vi "PSU Limit Check.vi"(8 "Error In":errorcluster, 10 "Supply Output":T1 {"Current mean" format="%.8f"; "Voltage mean" format="%.8f"; "Voltage min" format="%#_8g"; "Voltage max" format="%#_8g"; "Current min" format="%#_8g"; "Current max" format="%#_8g"}, 11 "Config Type":T2={"PSU"={"Current Lower (mA)"=0.0, "Current Upper (mA)"=0.0, "Voltage Lower (V)"=0.0, "Voltage Upper (V)"=0.0}, "Mic"={"Sensitivity (mV/Pa)"={"Lower"=0.0, "Upper"=0.0}, "THD (%)"={"Lower"=0.0, "Upper"=0.0}, "Freq Response"=[]}, "Power Supply"={"Channel Name"="1", "Source Delay (Sec)"=0.5, "Measurement:Sense"=1008, "voltage level"=0.0, "voltage level range"=20.0, "current limit"=0.02, "current limit range"=0.02, "resource name"="PSU"}, "Test Sweep"={"Input Settings"={"IEPE min time to settle [s]"=0.0, "Responce Channel Settings"={"DSA response channel settings"={"coupling"=10045, "enable IEPE excitation"=FALSE, "IEPE current [mA]"=4.0}, "response channel info"={"sensor sensitivity"=1000.0, "engineering units"=1, "dB reference"=1.0, "custom label"="EU", "weighting filter"=0, "pregain"=0.0}, "AI response settings"={"response channel"="SOUNDACQ/ai1", "max value [V]"=10.0, "min value [V]"=-10.0, "terminal configuration"=-1}}, "Stimulus Channel Settings"={"AI stimulus settings"={"stimulus channel"="SOUNDACQ/ai0", "max value [V]"=2.0, "min value [V]"=-2.0, "terminal configuration"=-1}, "DSA stimulus channel settings"={"coupling"=10045, "enable IEPE excitation"=TRUE, "IEPE current [mA]"=4.0}, "stimulus channel info"={"sensor sensitivity"=11.4, "engineering units"=2, "dB reference"=2e-05, "custom label"="EU", "weighting filter"=0, "pregain"=0.0}}}, "Output Settings"={"AO source settings"={"excitation channel"="SOUNDACQ/ao0", "max value [V]"=10.0, "min value [V]"=-10.0, "terminal configuration"=-1}}}} {"Test Sweep"."Output Settings"."AO source settings"."terminal configuration" items=["Default"=-1, "RSE"=10083, "Differential"=10106, "Pseudodifferential"=12529]; "Test Sweep"."Output Settings"."AO source settings"."min value [V]" format="%0.2f"; "Test Sweep"."Output Settings"."AO source settings"."max value [V]" format="%0.2f"; "Test Sweep"."Input Settings"."Stimulus Channel Settings"."stimulus channel info"."pregain" format="%.2f"; "Test Sweep"."Input Settings"."Stimulus Channel Settings"."stimulus channel info"."weighting filter" items=["Linear", "A-weighting", "B-weighting", "C-weighting", "ITU-R 468-4", "Dolby", "CCITT", "C-message", "Wb", "Wc", "Wd", "We", "Wf", "Wh", "Wj", "Wk", "Wm", "AES17 20 kHz lowpass", "AES17 40 kHz lowpass", "AES17 20 kHz highpass", "AES17 40 kHz highpass"]; "Test Sweep"."Input Settings"."Stimulus Channel Settings"."stimulus channel info"."dB reference" format="%^.1e"; "Test Sweep"."Input Settings"."Stimulus Channel Settings"."stimulus channel info"."engineering units" items=["custom..."=0, "V"=1, "A"=21, "C"=30, "pC"=31, "s"=32, "-"=29, "Pa"=2, "N"=20, "g"=3, "m/s^2"=4, "m/s"=5, "m"=6, "mm/s"=12, "mm"=13, "micron/s"=14, "micron"=15, "in/s^2"=7, "in/s"=8, "in"=9, "mil/s"=10, "mil"=11, "rad/s^2"=16, "rad/s"=17, "rad"=18, "deg/s^2"=26, "deg/s"=27, "deg"=28, "RPM"=22, "cycle/s^2"=23, "Hz"=24, "cycle"=25, "strain"=19]; "Test Sweep"."Input Settings"."Stimulus Channel Settings"."stimulus channel info"."sensor sensitivity" format="%#_5f"; "Test Sweep"."Input Settings"."Stimulus Channel Settings"."DSA stimulus channel settings"."IEPE current [mA]" format="%.1f"; "Test Sweep"."Input Settings"."Stimulus Channel Settings"."DSA stimulus channel settings"."coupling" items=["AC"=10045, "DC"=10050, "GND"=10066]; "Test Sweep"."Input Settings"."Stimulus Channel Settings"."AI stimulus settings"."terminal configuration" items=["Default"=-1, "RSE"=10083, "NRSE"=10078, "Differential"=10106, "Pseudodifferential"=12529]; "Test Sweep"."Input Settings"."Stimulus Channel Settings"."AI stimulus settings"."min value [V]" format="%.2f"; "Test Sweep"."Input Settings"."Stimulus Channel Settings"."AI stimulus settings"."max value [V]" format="%.2f"; "Test Sweep"."Input Settings"."Responce Channel Settings"."AI response settings"."terminal configuration" items=["Default"=-1, "RSE"=10083, "NRSE"=10078, "Differential"=10106, "Pseudodifferential"=12529]; "Test Sweep"."Input Settings"."Responce Channel Settings"."AI response settings"."min value [V]" format="%.2f"; "Test Sweep"."Input Settings"."Responce Channel Settings"."AI response settings"."max value [V]" format="%.2f"; "Test Sweep"."Input Settings"."Responce Channel Settings"."response channel info"."pregain" format="%.2f"; "Test Sweep"."Input Settings"."Responce Channel Settings"."response channel info"."weighting filter" items=["Linear", "A-weighting", "B-weighting", "C-weighting", "ITU-R 468-4", "Dolby", "CCITT", "C-message", "Wb", "Wc", "Wd", "We", "Wf", "Wh", "Wj", "Wk", "Wm", "AES17 20 kHz lowpass", "AES17 40 kHz lowpass", "AES17 20 kHz highpass", "AES17 40 kHz highpass"]; "Test Sweep"."Input Settings"."Responce Channel Settings"."response channel info"."dB reference" format="%^.1e"; "Test Sweep"."Input Settings"."Responce Channel Settings"."response channel info"."engineering units" items=["custom..."=0, "V"=1, "A"=21, "C"=30, "pC"=31, "s"=32, "-"=29, "Pa"=2, "N"=20, "g"=3, "m/s^2"=4, "m/s"=5, "m"=6, "mm/s"=12, "mm"=13, "micron/s"=14, "micron"=15, "in/s^2"=7, "in/s"=8, "in"=9, "mil/s"=10, "mil"=11, "rad/s^2"=16, "rad/s"=17, "rad"=18, "deg/s^2"=26, "deg/s"=27, "deg"=28, "RPM"=22, "cycle/s^2"=23, "Hz"=24, "cycle"=25, "strain"=19]; "Test Sweep"."Input Settings"."Responce Channel Settings"."response channel info"."sensor sensitivity" format="%#_5f"; "Test Sweep"."Input Settings"."Responce Channel Settings"."DSA response channel settings"."IEPE current [mA]" format="%.1f"; "Test Sweep"."Input Settings"."Responce Channel Settings"."DSA response channel settings"."coupling" items=["AC"=10045, "DC"=10050, "GND"=10066]; "Test Sweep"."Input Settings"."IEPE min time to settle [s]" format="%.1f"; "Power Supply"."current limit range" format="%_6p"; "Power Supply"."current limit" format="%_6p"; "Power Supply"."voltage level range" format="%_6p"; "Power Supply"."voltage level" format="%_6p"; "Power Supply"."Measurement:Sense" items=["Local"=1008, "Remote"=1009]; "Power Supply"."Source Delay (Sec)" format="%_6p"}) -> (0 "Error Out":errorcluster, 1 "PSU Result":bool, 3 "PSU":cluster{"Current (mA)":dbl, "Voltage (V)":dbl}, 5 "Current Result":bool, 7 "Volt Result":bool)   [LabVIEW 2018]
uses:
  Types/ME79 Specs.ctl
  <vilib>/addons/_NISVFA/_Shared subVIs/Controls/svc_DSA Channel Settings.ctl
  <vilib>/addons/_NISVFA/_Shared subVIs/Controls/svc_Channel Info.ctl
  <vilib>/addons/_NISVFA/_Shared subVIs/Controls/svc_Engineering Units Text Ring.ctl
  <vilib>/addons/_NISVFA/_Shared subVIs/Controls/svc_Weighting Filter Text Ring.ctl
  PowerSupply4110/Type/SupplyOutput.ctl
panel:
  # "Power Supply"
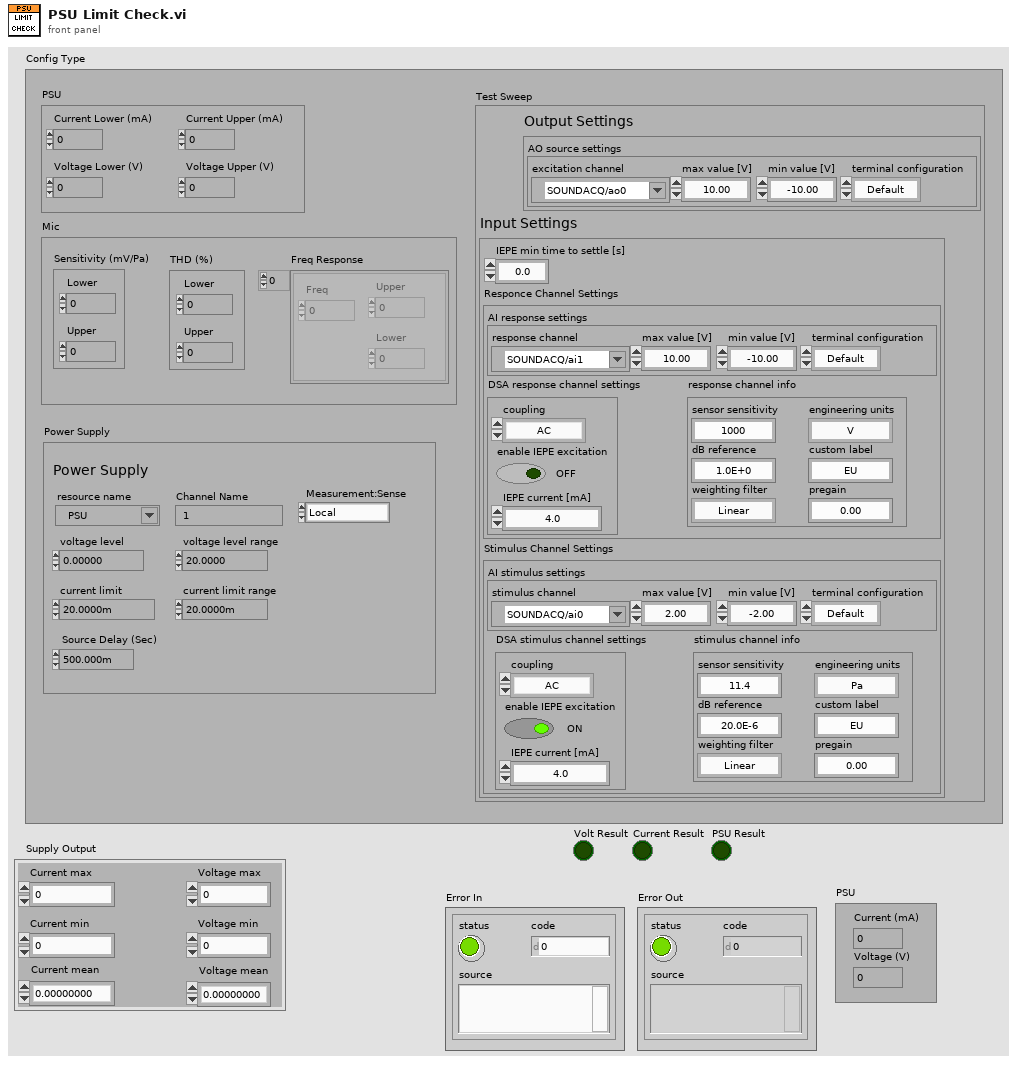
[diagram p1: front panel]
types:
  T1 = typedef "SupplyOutput.ctl" = cluster{"Current max":dbl, "Current min":dbl, "Voltage max":dbl, "Voltage min":dbl, "Voltage mean":dbl, "Current mean":dbl}
  T2 = typedef "ME79 Specs.ctl" = cluster{"PSU":cluster{"Current Lower (mA)":dbl, "Current Upper (mA)":dbl, "Voltage Lower (V)":dbl, "Voltage Upper (V)":dbl}, "Mic":cluster{"Sensitivity (mV/Pa)":cluster{"Lower":dbl, "Upper":dbl}, "THD (%)":cluster{"Lower":dbl, "Upper":dbl}, "Freq Response":cluster{"Freq":dbl, "Upper":dbl, "Lower":dbl}[]}, "Power Supply":cluster{"Channel Name":string, "Source Delay (Sec)":dbl, "Measurement:Sense":i32, "voltage level":dbl, "voltage level range":dbl, "current limit":dbl, "current limit range":dbl, "resource name":refnum<k15>}, "Test Sweep":cluster{"Input Settings":cluster{"IEPE min time to settle [s]":dbl, "Responce Channel Settings":cluster{"DSA response channel settings":T3, "response channel info":T4, "AI response settings":cluster{"response channel":tag, "max value [V]":dbl, "min value [V]":dbl, "terminal configuration":i32}}, "Stimulus Channel Settings":cluster{"AI stimulus settings":cluster{"stimulus channel":tag, "max value [V]":dbl, "min value [V]":dbl, "terminal configuration":i32}, "DSA stimulus channel settings":T3, "stimulus channel info":T4}}, "Output Settings":cluster{"AO source settings":cluster{"excitation channel":tag, "max value [V]":dbl, "min value [V]":dbl, "terminal configuration":i32}}}}
  T3 = typedef "svc_DSA Channel Settings.ctl" = cluster{"coupling":i32, "enable IEPE excitation":bool, "IEPE current [mA]":dbl}
  T4 = typedef "svc_Channel Info.ctl" = cluster{"sensor sensitivity":dbl, "engineering units":T5, "dB reference":dbl, "custom label":string, "weighting filter":T6, "pregain":dbl}
  T5 = typedef "svc_Engineering Units Text Ring.ctl" = u16
  T6 = typedef "svc_Weighting Filter Text Ring.ctl" = u16
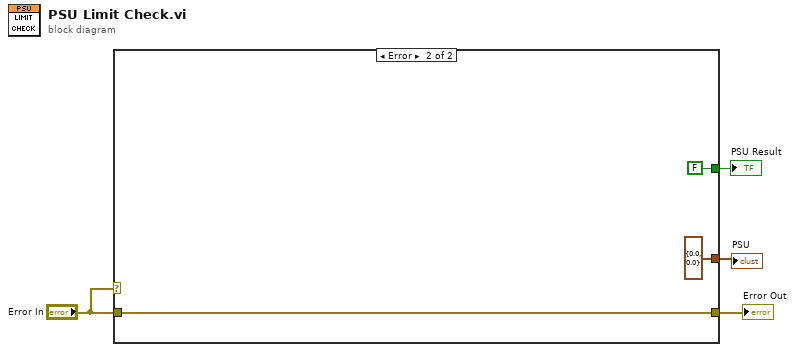
[diagram p0: block diagram]
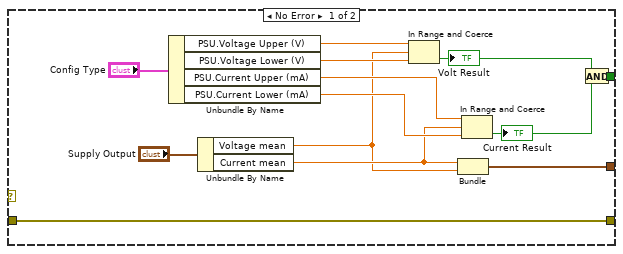
[diagram p2: hidden frame]
diagram:
  n1 = case shown="Error" "Error In" {
    tunnel: [w9 FALSE] -> w4
    tunnel: "Error In" -> [w8 w20]
    tunnel: [w8 w20] -> w2
    tunnel: [w5 cluster{"Current mean":dbl, "Voltage mean":dbl} {"Current mean"=0.0, "Voltage mean"=0.0}] -> w1
    frame No Error {
      n2 = Unbundle By Name("Config Type") -> ("PSU.Voltage Upper (V)"=w15:dbl, "PSU.Voltage Lower (V)"=w14:dbl, "PSU.Current Upper (mA)"=w13:dbl, "PSU.Current Lower (mA)"=w12:dbl)
      n3 = Unbundle By Name("Supply Output") -> ("Voltage mean"=w6:dbl, "Current mean"=w7:dbl)
      n4 = In Range and Coerce(upper limit=w15, x=w6, lower limit=w14) -> (In Range?=w11:bool)  [unwired: 1 out]
      "Volt Result" <- w11
      n5 = Bundle("Current mean"=w7, "Voltage mean"=w6) -> (w5:cluster{"Current mean":dbl, "Voltage mean":dbl})  [unwired: 1 in]
      n6 = In Range and Coerce(upper limit=w13, x=w7, lower limit=w12) -> (In Range?=w10:bool)  [unwired: 1 out]
      "Current Result" <- w10
      n7 = And(x=w11, y=w10) -> (x .and. y?=w9:bool)
    }
    frame Error {
    }
  }
  "PSU Result" <- w4
  "Error Out" <- w2
  "PSU" <- w1
